vi "TestErrorCorrection.vi"() -> ()   [LabVIEW 2010]
panel:
  out "Output Message":string
  out "Success":bool
  out "Encoded Output Message":u8[](array[numeric])
  in  "Use":bool
  in  "Test Message":u8[](array[numeric])
  out "Encoded Message":u8[](array[numeric])
  out "Original Message":u8[](array[numeric])
  in  "Input Message":string
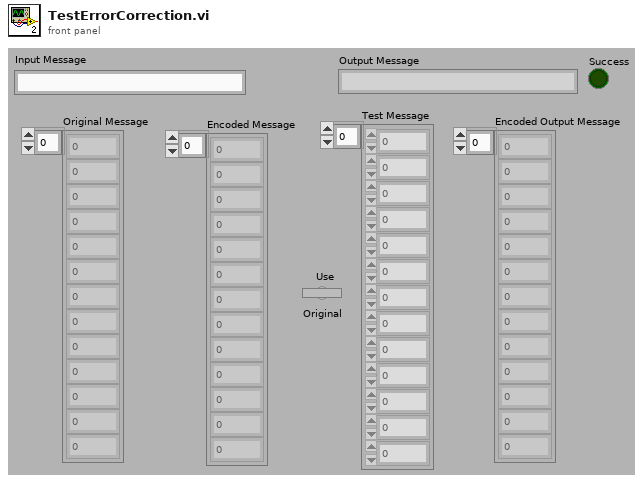
[diagram p1: front panel]
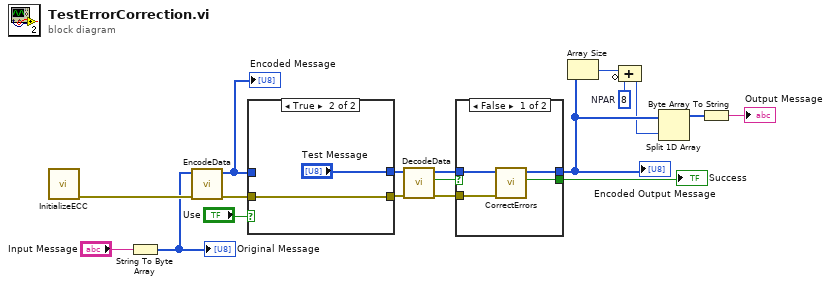
[diagram p0: block diagram]
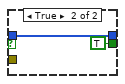
[diagram p2: hidden frame]
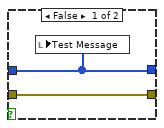
[diagram p3: hidden frame]
diagram:
  w5 = 8  # NPAR
  n1 = call "InitializeECC.vi"() -> ("Error Out"=w17:errorcluster)  [unwired: 11 in]
  n2 = String To Byte Array(string="Input Message") -> (unsigned byte array=w16:u8[])
  "Original Message" <- w16
  n3 = call "EncodeData.vi"("Error In"=w17, "Data In"=w16) -> ("Error Out"=w14:errorcluster, "Encoded Data Out"=w11:u8[])  [unwired: 8 in]
  "Encoded Message" <- w11
  n4 = case shown="True" "Use" {
    tunnel: w11 -> [w20 _]
    tunnel: w14 -> [w19 w21]
    tunnel: [w20 "Test Message"] -> w13
    tunnel: [w19 w21] -> w12
    frame False {
      n5 = local write "Test Message"(w20) -> ()
    }
    frame True {
    }
  }
  n6 = call "DecodeData.vi"("Error In"=w12, "Encoded Data"=w13) -> ("Error Out"=w8:errorcluster, "Check Syndrome"=w10:bool, "Encoded Data Out"=w9:u8[])  [unwired: 7 in]
  n7 = case shown="False" w10 {
    tunnel: w9 -> [w26 w28]
    tunnel: w8 -> [w25 _]
    tunnel: [w24 w28] -> w4
    tunnel: [w23 TRUE ("Success")] -> w7
    frame False {
      n8 = call "CorrectErrors.vi"("Error In"=w25, "Encoded Data"=w26) -> ("Success"=w23:bool, "Corrected Data"=w24:u8[])  [unwired: 7 in, 1 out]
    }
    frame True {
    }
  }
  "Encoded Output Message" <- w4
  "Success" <- w7
  n9 = Array Size(array=w4) -> (size(s)=w6:i32)
  n10 = Compound Arithmetic op=ADD(w6, invert w5) -> (w3:i32)
  n11 = Split 1D Array(array=w4, index=w3) -> (first subarray=w2:u8[])  [unwired: 1 out]
  n12 = Byte Array To String(unsigned byte array=w2) -> (string=→"Output Message":string)
